vi "Test Format LogRecord.vi"(8 "error in":errorcluster) -> (0 "error out":errorcluster)   [LabVIEW 2016, in "UT_Formatter.lvlib"]
doc: "Test the processing of an LogRecord."
uses:
  UT_Formatter.lvlib
  Source/HSE-Logger/LogLevel.ctl
  Source/HSE-Logger/LogRecord/LogRecord.lvclass/LogRecord.ctl
  Source/HSE-Logger/Handler/FileHandler/FileHandler.lvclass
  <vilib>/addons/_JKI Toolkits/Caraya/classes/Test/Test.lvclass
  Source/HSE-Logger/hse-logger.lvlib
  Source/HSE-Logger/LogRecord/LogRecord.lvclass
  Source/HSE-Logger/Formatter/Formatter.lvclass
  <vilib>/addons/_JKI Toolkits/Caraya/classes/Assert/Assert.lvclass
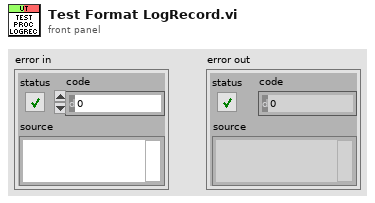
[diagram p1: front panel]
types:
  T1 = typedef "hse-logger.lvlib/LogLevel.ctl" = enum16{"DEBUG", "INFO", "WARNING", "ERROR", "CRITICAL"}
  T2 = enum16{"open", "replace", "create", "open or create", "replace or create", "replace or create with confirmation"}
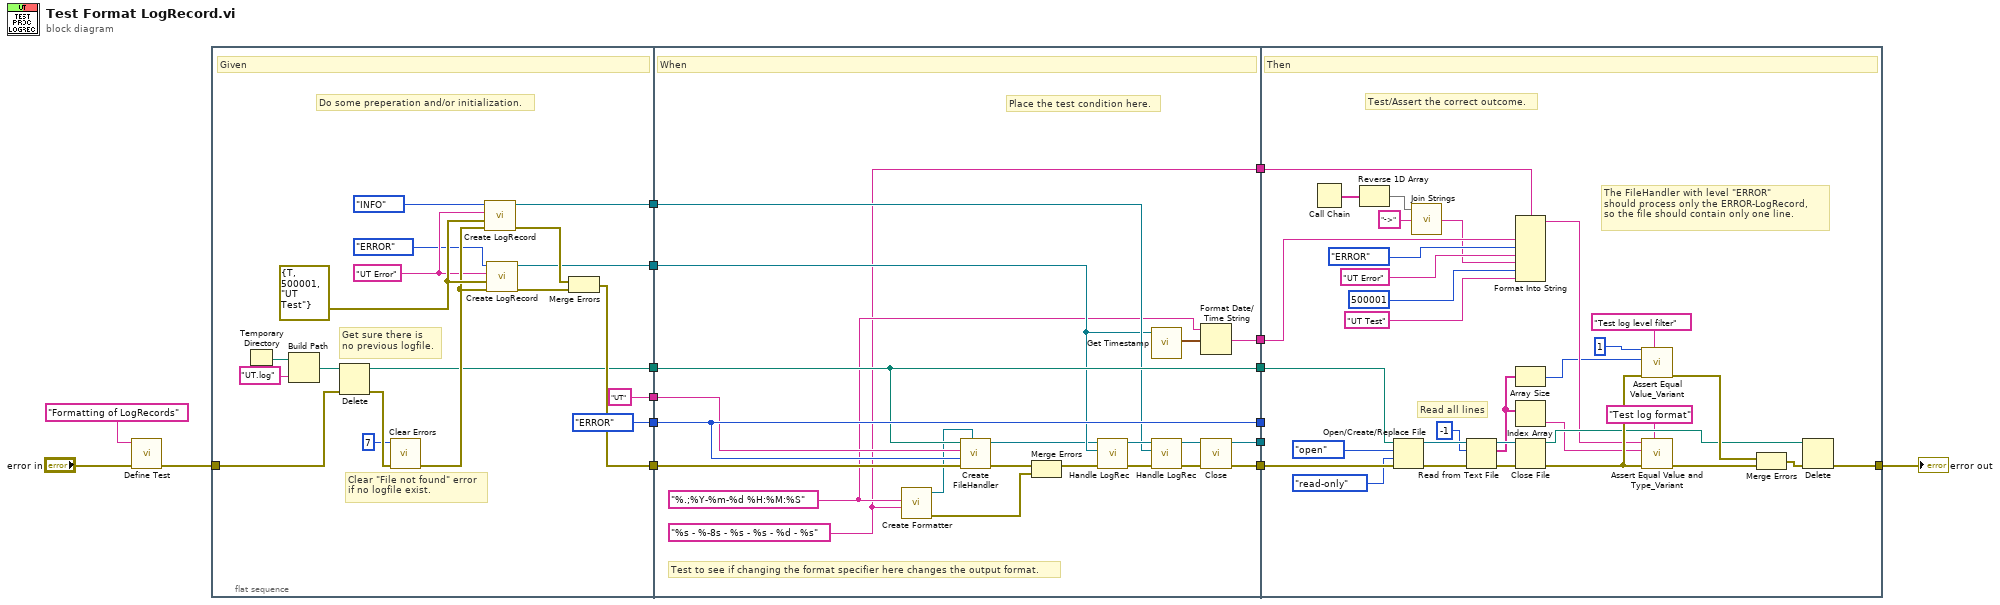
[diagram p0: block diagram]
diagram:
  n1 = call <vilib>:"Define Test.vi"("error in (no error)"="error in", "Label (VI Title)"="Formatting of LogRecords") -> ("error out"=w13:errorcluster)  [unwired: 8 in, 1 out]
  n2 = flat-sequence {
    tunnel: w13 -> [w35]
    tunnel: [w30] -> w16
    tunnel: [LogLevel."ERROR" ("Level")] -> w10
    tunnel: ["UT" ("Name")] -> w9
    tunnel: [w23] -> w8
    tunnel: [w21] -> w4
    tunnel: [w19] -> w3
    tunnel: w16 -> [w56]
    tunnel: [w55] -> w12
    tunnel: w10 -> [w50]
    tunnel: w9 -> [w49]
    tunnel: w8 -> [w48]
    tunnel: [w47] -> w7
    tunnel: [w50] -> w6
    tunnel: [w48] -> w5
    tunnel: w4 -> [w43]
    tunnel: w3 -> [w44]
    tunnel: [w40] -> w2
    tunnel: [w39] -> w1
    tunnel: [w82] -> w15
    tunnel: w12 -> [w87]
    tunnel: w7 -> [_]
    tunnel: w6 -> [_]
    tunnel: w5 -> [w80]
    tunnel: w2 -> [w65]
    tunnel: w1 -> [w64]
    frame #0 {
      w32 = errorcluster {"status"=TRUE, "code"=500001, "source"="UT Test"} ("Error to Log")
      w20 = "UT Error" ("Message")
      # "Clear \"File not found\" error\nif no logfile exist."
      # "Get sure there is\nno previous logfile."
      # "Do some preperation and/or initialization."
      # "Given"
      n3 = Temporary Directory() -> (w26:path)
      n4 = Build Path(base path=w26, name or relative path="UT.log") -> (appended path=w24:path)
      n5 = Delete(path (use dialog)=w24, error in=w35) -> (deleted path=w23:path, error out=w34:errorcluster)  [unwired: 3 in, 1 out]
      n6 = call <vilib>:"Clear Errors.vi"("error in (no error)"=w34, "specific error code to clear (0: all)"=7) -> ("error out"=w31:errorcluster)  [unwired: 4 in, 1 out]
      n7 = call "Create LogRecord.vi"("error in"=w31, "Error to Log"=w32, "Message"=w20, "Level"=LogLevel."INFO") -> ("error out"=w29:errorcluster, "LogRecord out"=w19:refnum<class "LogRecord.lvclass">)  [unwired: 6 in]
      n8 = call "Create LogRecord.vi"("error in"=w31, "Error to Log"=w32, "Message"=w20, "Level"=LogLevel."ERROR") -> ("error out"=w33:errorcluster, "LogRecord out"=w21:refnum<class "LogRecord.lvclass">)  [unwired: 6 in]
      n9 = Merge Errors(w29, w33) -> (w30:errorcluster)
    }
    frame #1 {
      w39 = "%s - %-8s - %s - %s - %d - %s" ("Format Specifier")
      w41 = "%.;%Y-%m-%d %H:%M:%S" ("Datetime format")
      # "Test to see if changing the format specifier here changes the output format."
      # "Place the test condition here."
      # "When"
      n10 = call "Create Formatter.vi"("Format Specifier"=w39, "Datetime format"=w41) -> ("error out"=w52:errorcluster, "Formatter out"=w36:refnum<class "Formatter.lvclass">)  [unwired: 8 in]
      n11 = call "Create FileHandler.vi"("Formatter.lvclass"=w36, "error in"=w56, "Level"=w50, "Name"=w49, "Filepath"=w48) -> ("error out"=w51:errorcluster, "FileHandler out"=w37:refnum<class "FileHandler.lvclass">)  [unwired: 5 in]
      n12 = Merge Errors(w51, w52) -> (w38:errorcluster)
      n13 = call-dynamic "Handle LogRec.vi"("error in"=w38, "LogRecord"=w43, "FileHandler in"=w37) -> ("error out"=w54:errorcluster, "FileHandler out"=w46:refnum<class "FileHandler.lvclass">)  [unwired: 7 in]
      n14 = call "Get Timestamp.vi"("LogRecord in"=w43) -> ("Created"=w42:timestamp)  [unwired: 8 in, 2 out]
      n15 = call-dynamic "Handle LogRec.vi"("error in"=w54, "LogRecord"=w44, "FileHandler in"=w46) -> ("error out"=w53:errorcluster, "FileHandler out"=w45:refnum<class "FileHandler.lvclass">)  [unwired: 7 in]
      n16 = Format Date/Time String(time format string (%c)=w41, seconds (now)=w42) -> (date/time string=w40:string)  [unwired: 1 in]
      n17 = call-dynamic "Close.vi"("error in"=w53, "FileHandler in"=w45) -> ("error out"=w55:errorcluster, "FileHandler out"=w47:refnum<class "FileHandler.lvclass">)  [unwired: 8 in]
    }
    frame #2 {
      # "The FileHandler with level \"ERROR\"\nshould process only the ERROR-LogRecord,\nso the file should contain only one line."
      # "Read all lines"
      # "Test/Assert the correct outcome."
      # "Then"
      n18 = Call Chain() -> (call chain=w58:string[])
      n19 = Reverse 1D Array(array=w58) -> (reversed array=w57:string[])
      n20 = Open/Create/Replace File(file path (use dialog)=w80, error in=w87, operation (0:open)=T2."open", access (0:read/write)=enum16{"read/write", "read-only", "write-only"}."read-only") -> (refnum out=w77:refnum<file>, error out=w86:errorcluster)  [unwired: 2 in, 1 out]
      n21 = call <vilib>:"Join Strings.vi"("Separator (,)"="->", "Strings In"=w57) -> ("String"=w61:string)  [unwired: 1 in]
      n22 = Read from Text File(file (use dialog)=w77, count=-1, error in=w86) -> (refnum out=w76:refnum<file>, text=w71:string[], error out=w84:errorcluster)  [unwired: 1 in, 1 out]
      n23 = Format Into String(format string=w64, w65, LogLevel."ERROR" ("Level"), "UT Error" ("Message"), w61, 500001 ("code"), "UT Test" ("Message")) -> (resulting string=w74:string)  [unwired: 2 in, 1 out]
      n24 = Array Size(array=w71) -> (size(s)=w69:i32)
      n25 = Index Array(array=w71) -> (element=w72:string)  [unwired: 1 in]
      n26 = Close File(refnum=w76, error in=w84) -> (path=w75:path, error out=w81:errorcluster)
      n27 = call <vilib>:"Assert Equal Value_Variant.vi"("Label"="Test log level filter", "error in (no error)"=w81, "Y"=w69, "X"=1 ("size(s)")) -> ("error out"=w88:errorcluster)  [unwired: 6 in, 1 out]
      n28 = call <vilib>:"Assert Equal Value and Type_Variant.vi"("Label"="Test log format", "error in (no error)"=w81, "Y"=w72, "X"=w74) -> ("error out"=w85:errorcluster)  [unwired: 6 in, 1 out]
      n29 = Merge Errors(w88, w85) -> (w83:errorcluster)
      n30 = Delete(path (use dialog)=w75, error in=w83) -> (error out=w82:errorcluster)  [unwired: 3 in, 2 out]
    }
  }
  "error out" <- w15
